vi "Populate Fault Channel Ring.vi"(11 "Fault Control":T1(array[cluster])) -> (3 "Array":string[](array[string]))   [LabVIEW 2013]
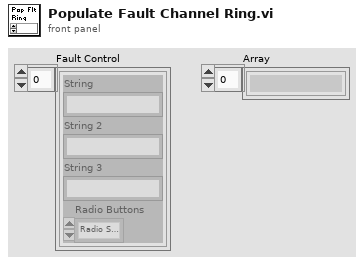
[diagram p1: front panel]
types:
  T1 = cluster{"String":string, "String 2":string, "String 3":string, "Radio Buttons":enum32{"Radio Selection 1", "Radio Selection 2", "Radio Selection 3", "Radio Selection 4", "Radio Selection 5"}}[]
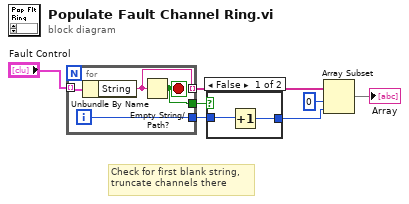
[diagram p0: block diagram]
diagram:
  # "Check for first blank string,\ntruncate channels there"
  n1 = for {
    tunnel: "Fault Control" -> [w11] mode=indexing
    tunnel: [w10] -> w2 mode=indexing
    tunnel: [w9] -> w6
    tunnel: [w8] -> w5
    i -> [w9]
    stop <- w8 stop-if-true
    n2 = Unbundle By Name(w11) -> ("String"=w10:string)
    n3 = Empty String/Path?(string/path=w10) -> (empty?=w8:bool)
  }
  n4 = case shown="False" w5 {
    tunnel: [w12 w14] -> w7
    tunnel: w6 -> [w13 w14]
    frame False {
      n5 = Increment(x=w13) -> (x+1=w12:i32)
    }
    frame True {
    }
  }
  n6 = Array Subset(array=w2, index=0, length=w7) -> (→"Array":string[])
